vi "Configure Arbitrary Waveform.vi"(4 "Frequency (1000 Hz)":dbl[unit]=1000.0, 6 "DC Offset (0 V)":dbl[unit], 7 "Arbitrary Waveform Name (0: USER1)":u16(ring) items=["USER1", "USER2", "USER3", "USER4"], 8 "error in (no error)":errorcluster, 9 "Gain (1 V)":dbl[unit]=1.0, 10 "Channel (0: Channel 1)":T1 items=["Channel 1", "Channel 2"], 11 "VISA resource name":refnum<visa-resource-name>) -> (0 "error out":errorcluster, 3 "VISA resource name out":refnum<visa-resource-name>)   [LabVIEW 2009, in "Tektronix AFG 3000 Series.lvlib"]
doc: "Configures the function generator settings that affect arbitrary waveform generation."
uses:
  Tektronix AFG 3000 Series.lvlib
  controls.llb/Channel.ctl
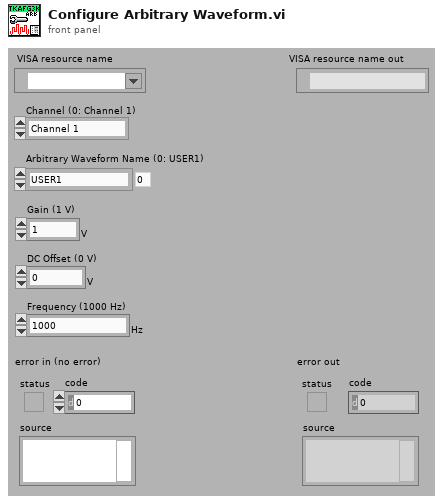
[diagram p1: front panel]
types:
  T1 = typedef "Channel.ctl" = u16
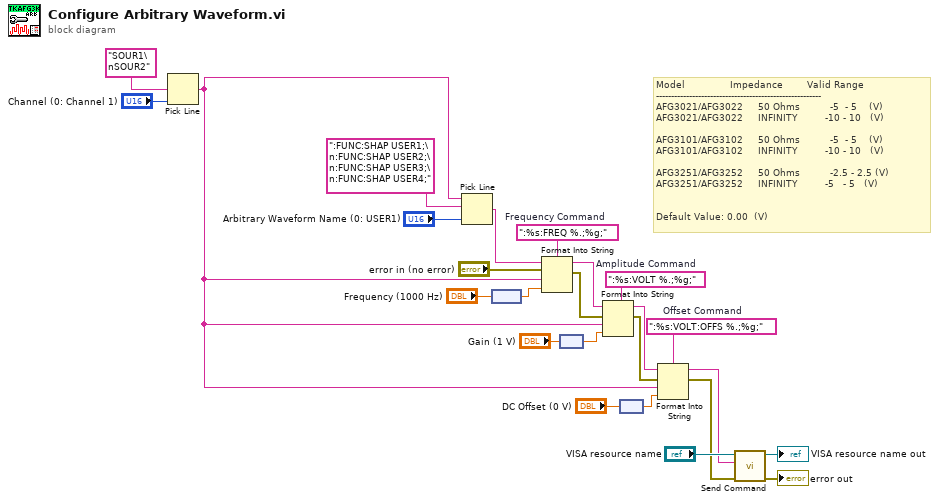
[diagram p0: block diagram]
diagram:
  w16 = ":%s:VOLT:OFFS %.;%g;"  # Offset Command
  w17 = ":%s:VOLT %.;%g;"  # Amplitude Command
  w18 = ":%s:FREQ %.;%g;"  # Frequency Command
  # "Model               Impedance        Valid Range\n-------------------------------------------------------\nAFG3021/AFG3022     50 Ohms          -5  - 5    (V)\nAFG3021/AFG3022     INFINITY         -10 - 10   (V)\n\nAFG3101/AFG3102     50 Ohms          -5  - 5    (V)\nAFG3101/AFG3102     INFINITY         -10 - 10   (V)\n\nAFG3251/AFG3252     50 Ohms          -2.5 - 2.5 (V)\nAFG3251/AFG3252     INFINITY         -5   - 5   (V)  \n\n\nDefault Value: 0.00  (V)"
  n1 = Pick Line(multi-line string="SOUR1\nSOUR2" ("string (\"\")"), line index="Channel (0: Channel 1)") -> (output string=w15:string)  [unwired: 1 out]
  n2 = Pick Line(string ("")=w15, multi-line string=":FUNC:SHAP USER1;\n:FUNC:SHAP USER2;\n:FUNC:SHAP USER3;\n:FUNC:SHAP USER4;" ("string (\"\")"), line index="Arbitrary Waveform Name (0: USER1)") -> (output string=w19:string)
  n3 = node("Frequency (1000 Hz)") -> (w10:dbl)
  n4 = Format Into String(format string=w18, initial string=w19, error in="error in (no error)", w15, w10) -> (resulting string=w23:string, error out=w13:errorcluster)
  n5 = node("Gain (1 V)") -> (w8:dbl)
  n6 = Format Into String(format string=w17, initial string=w23, error in=w13, w15, w8) -> (resulting string=w22:string, error out=w12:errorcluster)
  n7 = node("DC Offset (0 V)") -> (w6:dbl)
  n8 = Format Into String(format string=w16, initial string=w22, error in=w12, w15, w6) -> (resulting string=w4:string, error out=w3:errorcluster)
  n9 = call "Send Command.vi"("error in (no error)"=w3, "write buffer"=w4, "VISA resource name"="VISA resource name") -> ("error out"=→"error out":errorcluster, "VISA resource name out"=→"VISA resource name out":refnum<visa-resource-name>)  [unwired: 7 out]
